vi "source_config.vi"(8 "error in (no error)":errorcluster, 11 "Input parameters":T1={"Measurement type"=enum."Debug", "Sensor type"=enum."HPK_8in_271ch", "Identifier"="test.txt", "Open after execution?"=FALSE, "Plot after execution?"=FALSE, "Display channel"=0, "Voltage Delay (s)"=0.5, "Switch Delay (s)"=0.01, "VISA resource name source"="", "VISA resource name DMM"="", "VISA resource name LCR"="", "Compliance  Level (A)"=10.0, "Voltage Limit (V)"=1000.0, "Data storage location"="", "Scan voltages"="", "Use source as DMM?"=FALSE, "LCR signal frequenzy (Hz)"=10.0, "DMM device"=enum."Keithley2001", "Sampling number"=1, "Use env. sensors on"=enum."Sensirion sht1x/7x", "Switchboard Handle"=0, "Use Switchboard"=FALSE, "LCR signal voltage (V)"=10000.0, "Repeat"=1, "Scan voltages IV"="", "Scan voltages CV"="", "Hex pad numbers?"=FALSE, "Set measurement type"=enum."Debug", "Custom pad scan"="", "IV voltage Delay (s)"=0.5, "CV voltage Delay (s)"=0.5, "Needle measurement?"=FALSE, "Comments"="test.txt", "LCR signal frequenzy (kHz)"=10.0, "Compliance  Level (uA)"=10.0, "Open Correction Array"=array2304x3[6912 elements], "Current set voltage"=0.0, "Last set voltage"=0.0, "Current channel"=0, "Last OpenCorrection index"=-1, "Total curr/vltg every x steps"=10, "Current channel iteration"=0, "No CV corrections"=FALSE, "Mapfile"="", "Corrfile"="", "IV voltage file"=path "", "CV voltage file"=path "", "IV Switch Delay (s)"=0.01, "CV Switch Delay (s)"=0.01, "Invert polarity"=FALSE, "Set debug dirs"=FALSE, "Is n on p"=FALSE, "Source interlock?"=TRUE, "Voltage file used?"=FALSE, "Pad mask"="", "Mask pad above (uA)"=1.0, "LCR device"=enum."LCR_E4980", "Source device"=enum."Source_2410", "HexPlot binary path"="", "PadReductionFactor"=1.0, "Temperature degC"="", "Fluence [neq]"="", "Annealing [min]"=""} {"CV Switch Delay (s)" format="%#_13g"; "IV Switch Delay (s)" format="%#_13g"; "Last set voltage" format="%#_13g"; "Current set voltage" format="%#_13g"; "CV voltage Delay (s)" format="%#_13g"; "IV voltage Delay (s)" format="%#_13g"; "Voltage Limit (V)" format="%#_13g"; "Voltage Delay (s)" format="%#_13g"; "Switch Delay (s)" format="%#_13g"}) -> (0 "error out":errorcluster, 2 "Output Level (0)":dbl, 3 "VISA resource name out":refnum<visa-resource-name>)   [LabVIEW 2020]
doc: "Sets configuration for source meter."
uses:
  input_params.ctl
  <instrlib>/Keithley 24XX/Keithley 24XX.lvlib
  <instrlib>/Keithley 648X Series/Keithley 648X Series.lvlib
  <instrlib>/Keithley 2450/Keithley 2450.lvlib
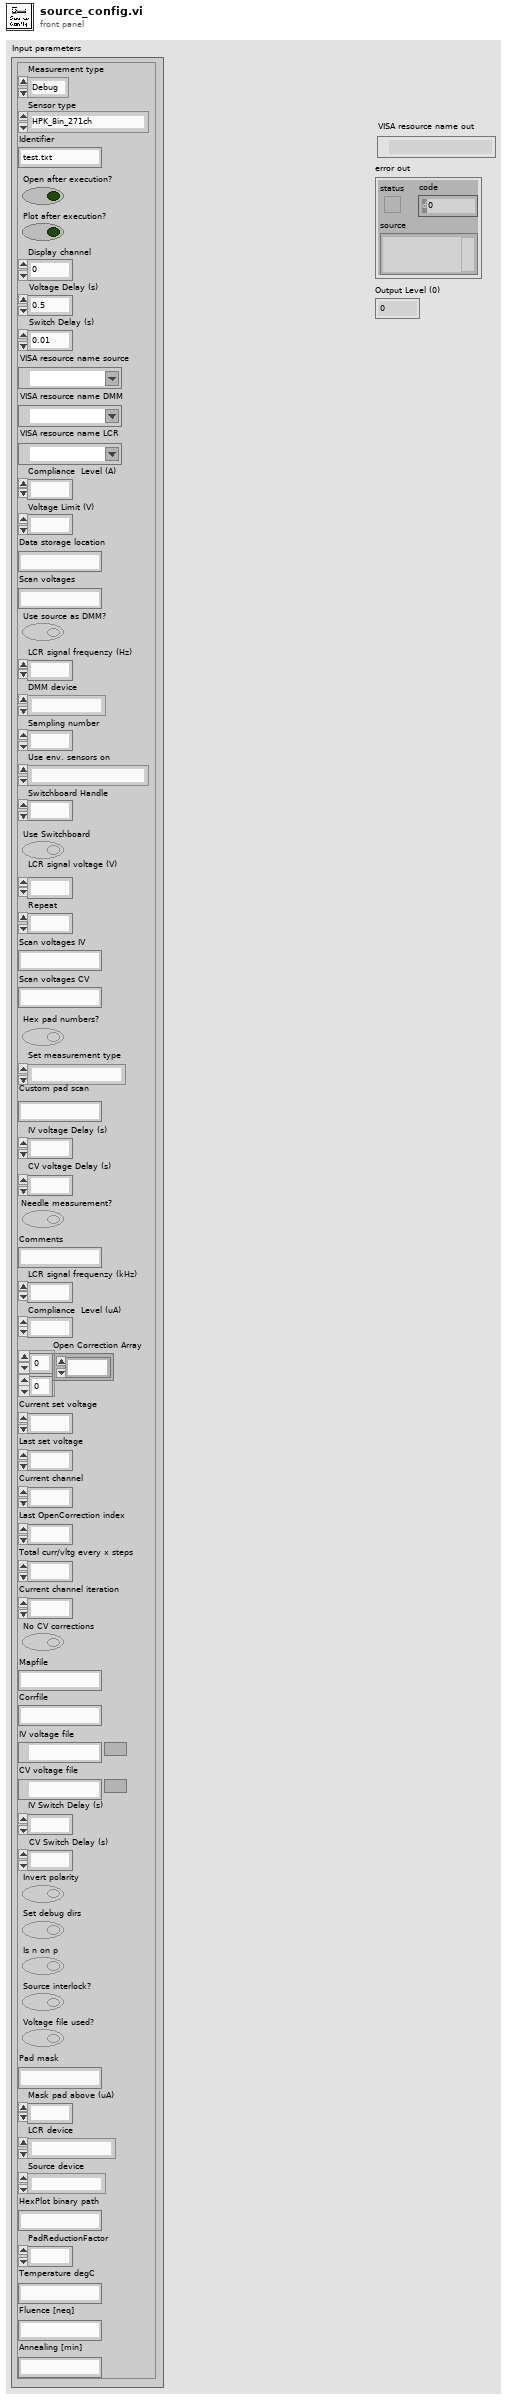
[diagram p1: front panel]
types:
  T1 = typedef "input_params.ctl" = cluster{"Measurement type":enum16{"IV", "CV", "Debug", "Test_contact"}, "Sensor type":enum16{"HPK_6in_135ch", "HPK_8in_271ch", "IFX_8in_256ch", "Diode", "HPK_6in_239ch", "Full_Matrix", "HPK_8in_271ch_full", "LumiCal", "HPK_8in_444ch", "HPK_8in_198ch_2019", "HPK_8in_MGW_LD_full", "HPK_8in_MGW_LD_a_type_top", "HPK_8in_MGW_LD_a_type_bottom", "HPK_8in_MGW_LD_b_type_left", "HPK_8in_MGW_LD_b_type_right", "HPK_8in_MGW_LD_c_type_left", "HPK_8in_MGW_LD_c_type_right", "HPK_8in_MGW_HD_full", "HPK_8in_MGW_HD_a_type_top", "HPK_8in_MGW_HD_a_type_bottom", "HPK_8in_MGW_HD_b_type_left", "HPK_8in_MGW_HD_b_type_right", "HPK_8in_MGW_HD_c_type_left", "HPK_8in_MGW_HD_c_type_right", "CALICE_6in_256ch"}, "Identifier":string, "Open after execution?":bool, "Plot after execution?":bool, "Display channel":i32, "Voltage Delay (s)":dbl, "Switch Delay (s)":dbl, "VISA resource name source":refnum<visa-resource-name>, "VISA resource name DMM":refnum<visa-resource-name>, "VISA resource name LCR":refnum<visa-resource-name>, "Compliance  Level (A)":dbl, "Voltage Limit (V)":dbl, "Data storage location":string, "Scan voltages":string, "Use source as DMM?":bool, "LCR signal frequenzy (Hz)":dbl, "DMM device":enum16{"Keithley2001", "Keithley2450", "Keithley2410", "Keithley6485", "Keithley6487", "Keithley6517"}, "Sampling number":i32, "Use env. sensors on":enum16{"Sensirion sht1x/7x", "Switch Matrix", "Probecard"}, "Switchboard Handle":u32, "Use Switchboard":bool, "LCR signal voltage (V)":dbl, "Repeat":i32, "Scan voltages IV":string, "Scan voltages CV":string, "Hex pad numbers?":bool, "Set measurement type":enum16{"IV", "CV", "Debug", "Test_contact", "IV+CV"}, "Custom pad scan":string, "IV voltage Delay (s)":dbl, "CV voltage Delay (s)":dbl, "Needle measurement?":bool, "Comments":string, "LCR signal frequenzy (kHz)":dbl, "Compliance  Level (uA)":dbl, "Open Correction Array":dbl[][], "Current set voltage":dbl, "Last set voltage":dbl, "Current channel":i32, "Last OpenCorrection index":i32, "Total curr/vltg every x steps":i32, "Current channel iteration":i32, "No CV corrections":bool, "Mapfile":string, "Corrfile":string, "IV voltage file":path, "CV voltage file":path, "IV Switch Delay (s)":dbl, "CV Switch Delay (s)":dbl, "Invert polarity":bool, "Set debug dirs":bool, "Is n on p":bool, "Source interlock?":bool, "Voltage file used?":bool, "Pad mask":string, "Mask pad above (uA)":dbl, "LCR device":enum16{"LCR_E4980", "AGILENT_4263X"}, "Source device":enum16{"Source_2410", "Source_6487", "Source_2470"}, "HexPlot binary path":string, "PadReductionFactor":dbl, "Temperature degC":string, "Fluence [neq]":string, "Annealing [min]":string}
  T2 = enum16{"Source_2410", "Source_6487", "Source_2470"}
  T3 = cluster{"Baud Rate":u32, "Parity":u16, "Data Bits":u16, "Stop Bits":u16, "Flow Control":u16}
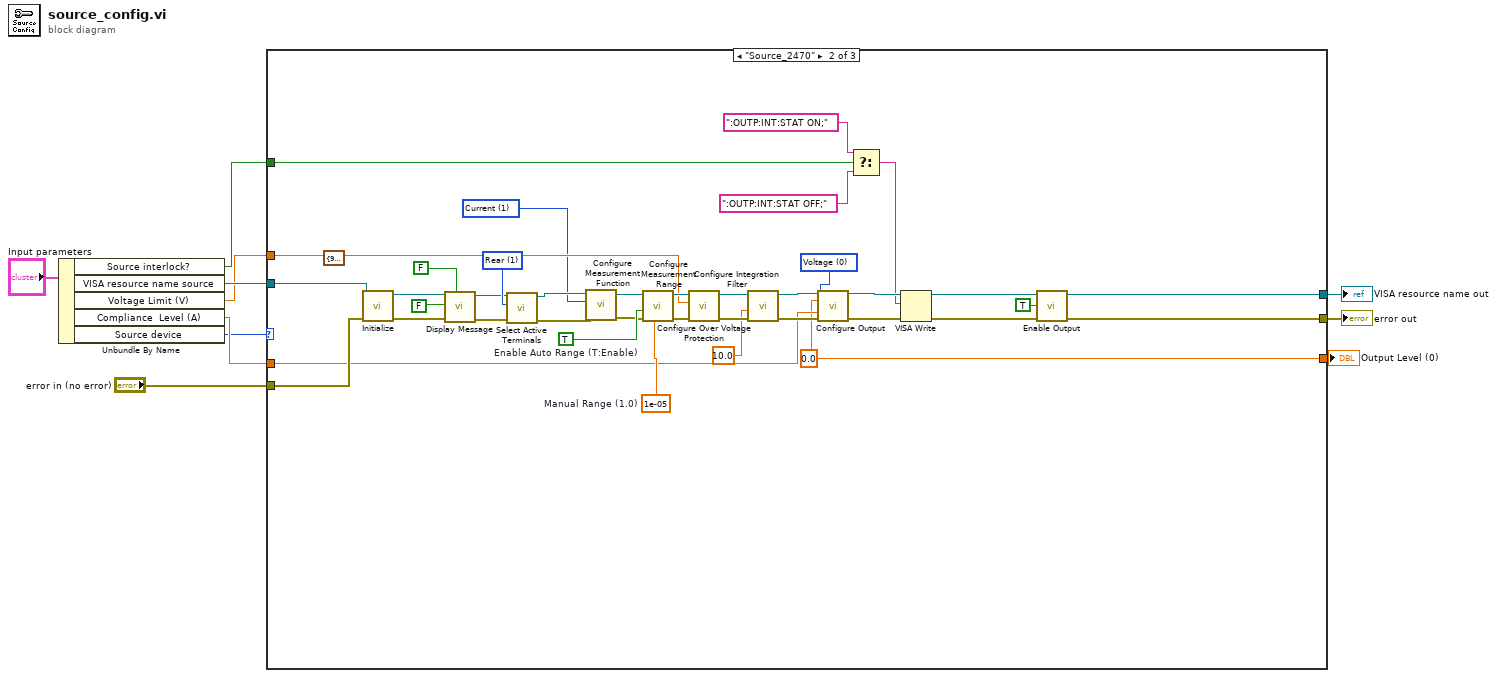
[diagram p0: block diagram]
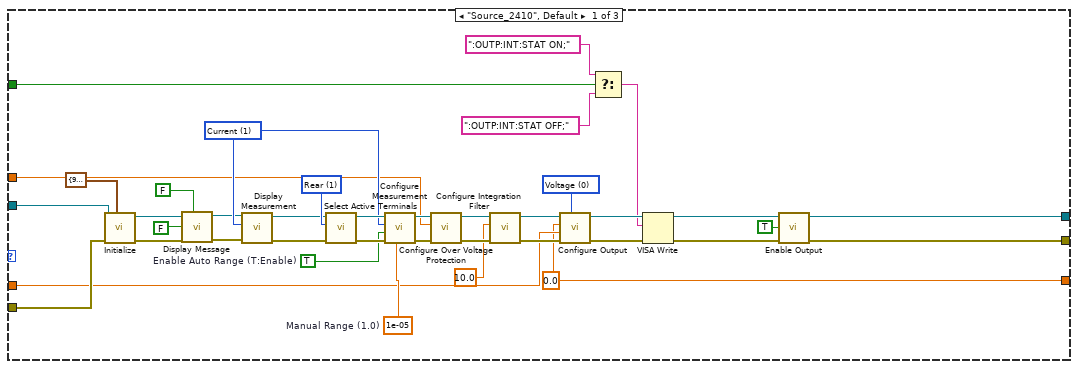
[diagram p2: hidden frame]
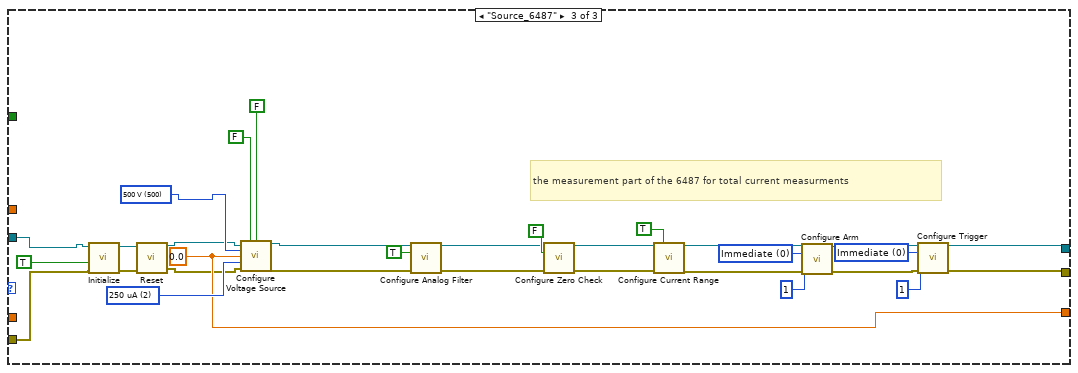
[diagram p3: hidden frame]
diagram:
  n1 = Unbundle By Name("Input parameters") -> ("Source interlock?"=w8:bool, "VISA resource name source"=w7:refnum<visa-resource-name>, "Voltage Limit (V)"=w6:dbl, "Compliance  Level (A)"=w5:dbl, "Source device"=w2:T2)
  n2 = case shown="\"Source_2470\"" w2 {
    tunnel: "error in (no error)" -> [w45 w84 w117]
    tunnel: w8 -> [w23 w67 _]
    tunnel: w7 -> [w19 w63 w118]
    tunnel: w6 -> [w18 w62 _]
    tunnel: w5 -> [w17 w61 _]
    tunnel: [w13 w57 w88] -> w4
    tunnel: [w14 w58 w89] -> w3
    tunnel: [w15 w59 w111] -> w1
    frame "Source_2410", Default {
      w33 = 1e-05  # Manual Range (1.0)
      w34 = TRUE  # Enable Auto Range (T:Enable)
      w32 = u16 1 items=["Voltage", "Current", "Resistance"] ("Displayed Measurement (0: Voltage)")
      w42 = u16 1 items=["Front", "Rear"] ("Active Terminals (0: Front)")
      w15 = 0.0 ("Output Level (0)")
      w48 = u16 0 items=["Voltage", "Current"] ("Source Mode  (0: Voltage)")
      n3 = call <instrlib>:"Initialize.vi"("Serial Configuration"=T3 {"Baud Rate"=9600, "Parity"=0, "Data Bits"=8, "Stop Bits"=10, "Flow Control"=0}, "error in (no error)"=w45, "VISA resource name"=w19) -> ("error out"=w30:errorcluster, "VISA resource name out"=w31:refnum<visa-resource-name>)  [unwired: 7 in]
      n4 = call <instrlib>:"Display Message.vi"("Enable Lower Message (T: Enable)"=FALSE, "Enable Upper Message (T: Enable)"=FALSE, "error in (no error)"=w30, "VISA resource name"=w31) -> ("error out"=w29:errorcluster, "VISA resource name out"=w28:refnum<visa-resource-name>)  [unwired: 6 in]
      n5 = call <instrlib>:"Display Measurement.vi"("error in (no error)"=w29, "Displayed Measurement (0: Voltage)"=w32, "VISA resource name"=w28) -> ("error out"=w41:errorcluster, "VISA resource name out"=w40:refnum<visa-resource-name>)  [unwired: 7 in]
      n6 = call <instrlib>:"Select Active Terminals.vi"("error in (no error)"=w41, "Active Terminals (0: Front)"=w42, "VISA resource name"=w40) -> ("error out"=w43:errorcluster, "VISA resource name out"=w44:refnum<visa-resource-name>)  [unwired: 7 in]
      n7 = call <instrlib>:"Configure Measurement.vi"("Manual Range (1.0)"=w33, "error in (no error)"=w43, "Enable Auto Range (T:Enable)"=w34, "Function (0: Volts)"=w32, "VISA resource name"=w44) -> ("error out"=w46:errorcluster, "VISA resource name out"=w47:refnum<visa-resource-name>)  [unwired: 5 in]
      n8 = call <instrlib>:"Configure Over Voltage Protection.vi"("error in (no error)"=w46, "Voltage Limit (0.0 V)"=w18, "VISA resource name"=w47) -> ("error out"=w38:errorcluster, "VISA resource name out"=w39:refnum<visa-resource-name>)  [unwired: 7 in]
      n9 = call <instrlib>:"Configure Integration Filter.vi"("error in (no error)"=w38, "Measurement Speed (1 PLC)"=10.0, "VISA resource name"=w39) -> ("error out"=w37:errorcluster, "VISA resource name out"=w36:refnum<visa-resource-name>)  [unwired: 7 in]
      n10 = call <instrlib>:"Configure Output.vi"("Source Mode  (0: Voltage)"=w48, "error in (no error)"=w37, "Compliance  Level (0.1)"=w17, "Output Level (0)"=w15, "VISA resource name"=w36) -> ("error out"=w25:errorcluster, "VISA resource name out"=w24:refnum<visa-resource-name>)  [unwired: 5 in]
      n11 = Select(t=":OUTP:INT:STAT ON;" ("write buffer"), s=w23, f=":OUTP:INT:STAT OFF;" ("write buffer")) -> (s? t:f=w20:string)
      n12 = VISA Write(VISA resource name=w24, write buffer=w20, error in (no error)=w25) -> (VISA resource name out=w12:refnum<visa-resource-name>, error out=w11:errorcluster)  [unwired: 1 out]
      n13 = call <instrlib>:"Enable Output.vi"("error in (no error)"=w11, "Enable Output (T: Enable)"=TRUE ("Enable Output"), "VISA resource name"=w12) -> ("error out"=w13:errorcluster, "VISA resource name out"=w14:refnum<visa-resource-name>)  [unwired: 7 in]
    }
    frame "Source_2470" {
      (unwired) T3 {"Baud Rate"=9600, "Parity"=0, "Data Bits"=8, "Stop Bits"=10, "Flow Control"=0} ("Serial Configuration")
      w76 = 1e-05  # Manual Range (1.0)
      w77 = TRUE  # Enable Auto Range (T:Enable)
      w50 = u16 1 items=["Voltage", "Current", "Resistance"] ("Displayed Measurement (0: Voltage)")
      w83 = u16 1 items=["Front", "Rear"] ("Active Terminals (0: Front)")
      w59 = 0.0 ("Output Level (0)")
      w87 = u16 0 items=["Voltage", "Current"] ("Source Mode  (0: Voltage)")
      n14 = call <instrlib>:"Initialize.vi"("error in (no error)"=w84, "VISA resource name"=w63) -> ("error out"=w74:errorcluster, "VISA resource name out"=w75:refnum<visa-resource-name>)  [unwired: 8 in]
      n15 = call <instrlib>:"Display Message.vi"("Enable Lower Message (T: Enable)"=FALSE, "Enable Upper Message (T: Enable)"=FALSE, "error in (no error)"=w74, "VISA resource name"=w75) -> ("error out"=w73:errorcluster, "VISA resource name out"=w72:refnum<visa-resource-name>)  [unwired: 6 in]
      n16 = call <instrlib>:"Select Active Terminals.vi"("error in (no error)"=w73, "Active Terminals (0: Front)"=w83, "VISA resource name"=w72) -> ("error out"=w54:errorcluster, "VISA resource name out"=w52:refnum<visa-resource-name>)  [unwired: 7 in]
      n17 = call <instrlib>:"Configure Measurement Function.vi"("error in (no error)"=w54, "Function (0: Volts)"=w50, "VISA resource name"=w52) -> ("error out"=w53:errorcluster, "VISA resource name out"=w51:refnum<visa-resource-name>)  [unwired: 7 in]
      n18 = call <instrlib>:"Configure Measurement Range.vi"("Manual Range (1.0)"=w76, "error in (no error)"=w53, "Enable Auto Range (T:Enable)"=w77, "VISA resource name"=w51) -> ("error out"=w85:errorcluster, "VISA resource name out"=w86:refnum<visa-resource-name>)  [unwired: 6 in]
      n19 = call <instrlib>:"Configure Over Voltage Protection.vi"("error in (no error)"=w85, "Voltage Limit (0)"=w62, "VISA resource name"=w86) -> ("error out"=w81:errorcluster, "VISA resource name out"=w82:refnum<visa-resource-name>)  [unwired: 7 in]
      n20 = call <instrlib>:"Configure Integration Filter.vi"("error in (no error)"=w81, "Measurement Speed (1 PLC)"=10.0, "VISA resource name"=w82) -> ("error out"=w80:errorcluster, "VISA resource name out"=w79:refnum<visa-resource-name>)  [unwired: 7 in]
      n21 = call <instrlib>:"Configure Output.vi"("VISA resource name"=w79, "Source Level (0)"=w59, "Source Mode  (0: Voltage)"=w87, "Source Limit Level (0.1)"=w61, "error in (no error)"=w80) -> ("VISA resource name out"=w68:refnum<visa-resource-name>, "error out"=w69:errorcluster)  [unwired: 9 in]
      n22 = Select(t=":OUTP:INT:STAT ON;" ("write buffer"), s=w67, f=":OUTP:INT:STAT OFF;" ("write buffer")) -> (s? t:f=w64:string)
      n23 = VISA Write(VISA resource name=w68, write buffer=w64, error in (no error)=w69) -> (VISA resource name out=w56:refnum<visa-resource-name>, error out=w55:errorcluster)  [unwired: 1 out]
      n24 = call <instrlib>:"Enable Output.vi"("error in (no error)"=w55, "Enable Output (T: Enable)"=TRUE ("Enable Output"), "VISA resource name"=w56) -> ("error out"=w57:errorcluster, "VISA resource name out"=w58:refnum<visa-resource-name>)  [unwired: 7 in]
    }
    frame "Source_6487" {
      w97 = u16 0 items=["Immediate", "Tlink"] ("Trigger Source (0: Immediate)")
      w99 = u16 0 items=["Immediate", "Timer", "Bus", "Tlink", "Manual", "Negative SOT", "Positive SOT", "Bidirectional SOT"] ("Arm Source (0: Immediate)")
      w111 = 0.0 ("Voltage Level (0 V)")
      w114 = u16 2 items=["25 mA", "2.5 mA", "250 uA", "25 uA"] ("Current Limit (25 mA)")
      w115 = u16 500 items=["10 V"=10, "50 V"=50, "500 V"=500] ("Voltage Source Range (10 V)")
      # "the measurement part of the 6487 for total current measurments"
      n25 = call <instrlib>:"Initialize.vi"("error in (no error)"=w117, "Reset (True)"=TRUE, "VISA resource name"=w118) -> ("error out"=w94:errorcluster, "VISA resource name out"=w95:refnum<visa-resource-name>)  [unwired: 7 in]
      n26 = call <instrlib>:"Reset.vi"("VISA resource name"=w95, "error in (no error)"=w94) -> ("VISA resource name out"=w93:refnum<visa-resource-name>, "error out"=w92:errorcluster)  [unwired: 12 in]
      n27 = call <instrlib>:"Configure Voltage Source.vi"("VISA resource name"=w93, "Enable Voltage Source (F: Disable)"=FALSE, "Enable Interlock (F: Disable)"=FALSE, "Voltage Source Range (10 V)"=w115, "Voltage Level (0 V)"=w111, "Current Limit (25 mA)"=w114, "error in (no error)"=w92) -> ("VISA resource name out"=w110:refnum<visa-resource-name>, "error out"=w109:errorcluster)  [unwired: 7 in]
      n28 = call <instrlib>:"Configure Analog Filter.vi"("VISA resource name"=w110, "Enable Damping Filter (T: Enable)"=TRUE, "error in (no error)"=w109) -> ("VISA resource name out"=w91:refnum<visa-resource-name>, "error out"=w90:errorcluster)  [unwired: 11 in]
      n29 = call <instrlib>:"Configure Zero Check.vi"("VISA resource name"=w91, "Enable Zero Check (T: Enable)"=FALSE ("Autozero"), "error in (no error)"=w90) -> ("VISA resource name out"=w105:refnum<visa-resource-name>, "error out"=w104:errorcluster)  [unwired: 11 in]
      n30 = call <instrlib>:"Configure Current Range.vi"("VISA resource name"=w105, "Autorange (T: Enable)"=TRUE, "error in (no error)"=w104) -> ("VISA resource name out"=w103:refnum<visa-resource-name>, "error out"=w100:errorcluster)  [unwired: 11 in]
      n31 = call <instrlib>:"Configure Arm.vi"("VISA resource name"=w103, "Arm Source (0: Immediate)"=w99, "Arm Loop Count (1)"=1, "error in (no error)"=w100) -> ("VISA resource name out"=w102:refnum<visa-resource-name>, "error out"=w101:errorcluster)  [unwired: 10 in]
      n32 = call <instrlib>:"Configure Trigger.vi"("VISA resource name"=w102, "Trigger Source (0: Immediate)"=w97, "Trigger Loop Count (1)"=1, "error in (no error)"=w101) -> ("VISA resource name out"=w89:refnum<visa-resource-name>, "error out"=w88:errorcluster)  [unwired: 10 in]
    }
  }
  "VISA resource name out" <- w3
  "error out" <- w4
  "Output Level (0)" <- w1
